vi "WPI_UtilitiesFRCAutomaticValuePublisher.vi"(11 "Enable":bool=TRUE) -> ()   [LabVIEW 2012]
uses:
  <vilib>/Rock Robotics/WPI/Utilities/Refnum Registry Operation.ctl
  <vilib>/Rock Robotics/WPI/Relay/WPI_RelayValue.ctl
  <vilib>/Rock Robotics/WPI/Solenoid/WPI_SolenoidValue.ctl
  <vilib>/Rock Robotics/WPI/Solenoid/WPI_SolenoidChannel.ctl
  <vilib>/Rock Robotics/WPI/Solenoid/WPI_SolenoidSetEnum.vi
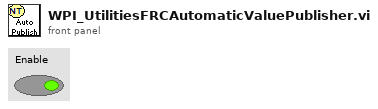
[diagram p1: front panel]
types:
  T1 = typedef "Refnum Registry Operation.ctl" = enum16{"set", "get", "delete", "get all names", "read name"}
  T2 = typedef "WPI_RelayValue.ctl" = enum16{"Off", "On", "Forward", "Reverse"}
  T3 = typedef "WPI_SolenoidChannel.ctl" = enum8{"Solenoid 1", "Solenoid 2", "Solenoid 3", "Solenoid 4", "Solenoid 5", "Solenoid 6", "Solenoid 7", "Solenoid 8", "Invalid"}
  T4 = typedef "WPI_SolenoidValue.ctl" = enum16{"Off", "On", "Forward", "Reverse"}
  T5 = typedef "WPI_JoystickDevRef.ctl" = cluster{"Device":T6}
  T6 = typedef "WPI_JoystickDeviceEnum.ctl" = enum16{"USB 1", "USB 2", "USB 3", "USB 4", "Kinect 1", "Kinect 2"}
  T7 = typedef "WPI_JoystickButtonState.ctl" = cluster{"Button 1":bool, "Button 2":bool, "Button 3":bool, "Button 4":bool, "Button 5":bool, "Button 6":bool, "Button 7":bool, "Button 8":bool, "Button 9":bool, "Button 10":bool, "Button 11":bool, "Button 12":bool}
  T8 = cluster{"axis 1 (x)":dbl, "axis 2 (y)":dbl, "axis 3 (throttle)":dbl, "axis 4":dbl, "axis 5":dbl, "axis 6":dbl}
  T9 = typedef "WPI_MotorControlDeviceRef.ctl" = cluster{"DeviceStatus":errorcluster, "Type":enum16{"PWM", "CAN"}, "PWM":cluster{"Digital Module":T10, "PWM Channel":T11, "DeadBand":T12}, "CAN":cluster{"Device Number":u8, "Control Mode":T13, "Semaphore":T14, "Max Vout":dbl}, "Invert":bool, "TransformRef":T15, "InvTransformRef":T15}
  T10 = typedef "FPGA_TypedefDigitalModule.ctl" = enum16{"Digital Module 1", "Digital Module 2"}
  T11 = typedef "FPGA_DIOPWMChannel.ctl" = enum8{"PWM 1", "PWM 2", "PWM 3", "PWM 4", "PWM 5", "PWM 6", "PWM 7", "PWM 8", "PWM 9", "PWM 10", "Invalid"}
  T12 = typedef "WPI_PWMDeadband.ctl" = cluster{"Name":string, "maxPositivePwm":i32, "minPositivePwm":i32, "centerPwm":i32, "maxNegativePwm":i32, "minNegativePwm":i32, "angularRange":u16}
  T13 = typedef "WPI_CANJaguar_ControlMode.ctl" = enum8{"Percent VBus", "Current", "Speed", "Position", "Voltage"}
  T14 = typedef "Semaphore RefNum" = refnum<k1>
  T15 = typedef "WPI_PWMTransform_ConPane.ctl" = refnum<vi>
  T16 = typedef "WPI_ServoDeviceRef.ctl" = cluster{"DeviceStatus":errorcluster, "Digital Module":T10, "PWM Channel":T11, "DeadBand":T12}
  T17 = typedef "WPI_RelayDevRef.ctl" = cluster{"DevStatus":errorcluster, "Relay Channel":T18, "Digital Module":T10, "Relay Direction":T19}
  T18 = typedef "FPGA_DIORelayChannel.ctl" = enum8{"Relay 1", "Relay 2", "Relay 3", "Relay 4", "Relay 5", "Relay 6", "Relay 7", "Relay 8", "Invalid"}
  T19 = typedef "WPI_RelayDirection.ctl" = enum16{"Both directions", "Forward only", "Reverse only"}
  T20 = typedef "WPI_CompressorDevRef.ctl" = cluster{"DevStatus":errorcluster, "DigitalInputDevRef":T21, "RelayDevRef":T17}
  T21 = typedef "WPI_DigitalInputDevRef.ctl" = cluster{"DevStatus":errorcluster, "DIO Channel":T22, "Digital Module":T10}
  T22 = typedef "FPGA_DIOChannel.ctl" = enum8{"DIO 1", "DIO 2", "DIO 3", "DIO 4", "DIO 5", "DIO 6", "DIO 7", "DIO 8", "DIO 9", "DIO 10", "DIO 11", "DIO 12", "DIO 13", "DIO 14", "Invalid"}
  T23 = typedef "WPI_SolenoidDevRef.ctl" = cluster{"DevStatus":errorcluster, "Solenoid Module":T24, "Forward Solenoid Channel":T3, "Reverse Solenoid Channel":T3}
  T24 = typedef "FPGA_TypedefSolenoidModule.ctl" = enum16{"Solenoid Module 1", "Solenoid Module 2"}
  T25 = typedef "WPI_AccelerometerDevRef.ctl" = cluster{"DevStatus":errorcluster, "Analog Module":T26, "Analog Channel":T27, "Scaling":T28}
  T26 = typedef "FPGA_TypedefAnalogModule.ctl" = enum16{"Analog Module 1", "Analog Module 2"}
  T27 = typedef "FPGA_AIChannel.ctl" = enum8{"AI 1", "AI 2", "AI 3", "AI 4", "AI 5", "AI 6", "AI 7", "AI 8", "Invalid"}
  T28 = typedef "WPI_AccelerometerScaling.ctl" = cluster{"Gain (VoltsPerG)":dbl, "Center Voltage":dbl}
  T29 = typedef "WPI_CounterDevRef.ctl" = cluster{"DevStatus":errorcluster, "CntIndex":T30}
  T30 = typedef "FPGA_CounterCtrSystemIndex.ctl" = enum8{"Ctr 0", "Ctr 1", "Ctr 2", "Ctr 3", "Ctr 4", "Ctr 5", "Ctr 6", "Ctr 7", "Invalid"}
  T31 = typedef "WPI_GyroDevRef.ctl" = cluster{"DevStatus":errorcluster, "Analog Module":T26, "Analog Channel":T27, "Offset":dbl, "Gain (VoltsPerDegree/Second)":dbl}
  T32 = typedef "WPI_UltrasonicDeviceRef.ctl" = cluster{"DevStatus":errorcluster, "Ping Digital Module":T10, "Echo Digital Module":T10, "Ping Channel":T22, "Echo Channel":T22, "CntIndex":T30}
  T33 = typedef "WPI_EncoderDevRef.ctl" = cluster{"DevStatus":errorcluster, "EncoderIndex":T34, "CounterIndex":T30, "DistancePerCount":dbl, "Decoding Type":T35}
  T34 = typedef "FPGA_EncoderIdx.ctl" = enum8{"Enc 0", "Enc 1", "Enc 2", "Enc 3", "Invalid"}
  T35 = typedef "WPI_EncoderType.ctl" = enum16{"1x", "2x", "4x"}
  T36 = typedef "WPI_DigitalOutputDevRef.ctl" = cluster{"Digital Module":T10, "DIO Channel":T22, "DevStatus":errorcluster}
  T37 = typedef "WPI_PWMDeviceRef.ctl" = cluster{"DeviceStatus":errorcluster, "Digital Module":T10, "PWM Channel":T11}
  T38 = typedef "WPI_AnalogChannelDevRef.ctl" = cluster{"DevStatus":errorcluster, "Analog Module":T26, "Analog Channel":T27}
  T39 = typedef "WPI_CameraDevRef.ctl" = cluster{"Camera Address":string, "CameraStatus":errorcluster, "Acquire Image Notifier":refnum<notifier>}
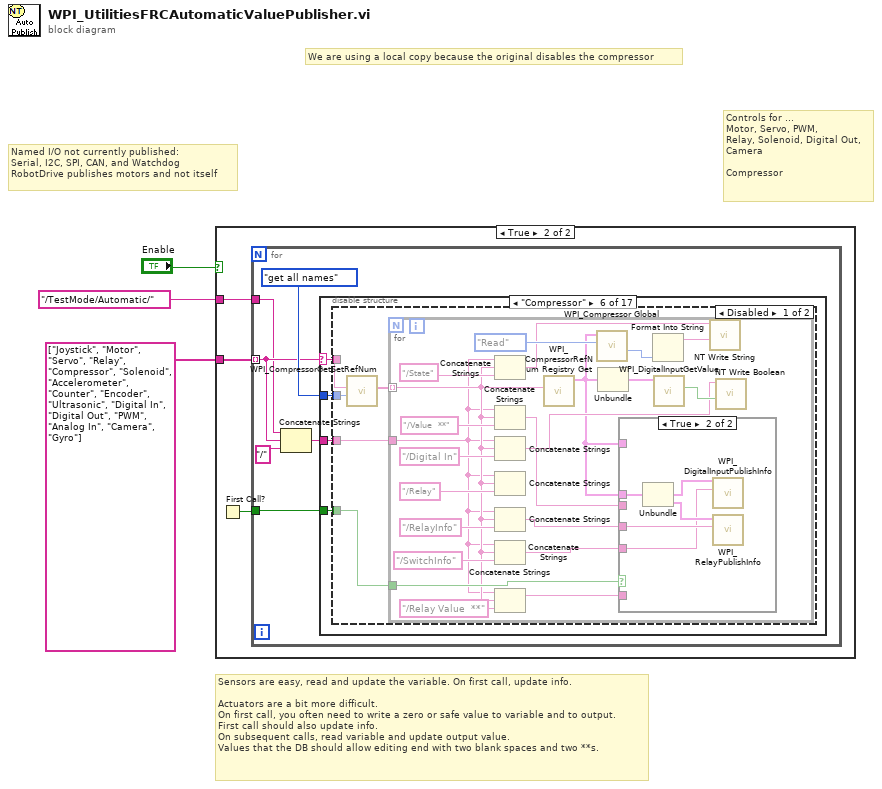
[diagram p0: block diagram]
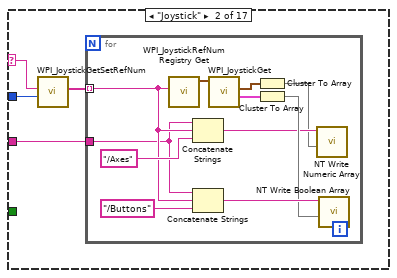
[diagram p4: hidden frame]
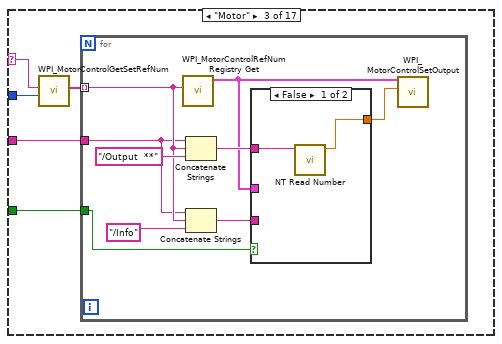
[diagram p5: hidden frame]
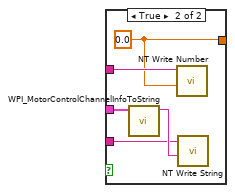
[diagram p6: hidden frame]
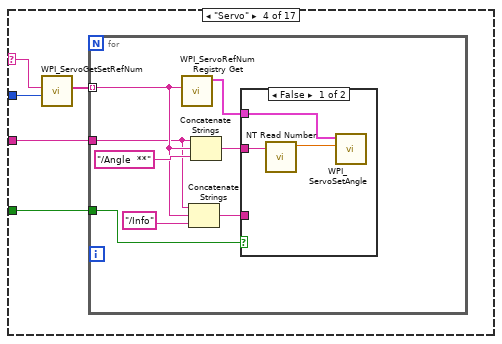
[diagram p7: hidden frame]
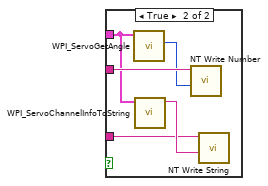
[diagram p8: hidden frame]
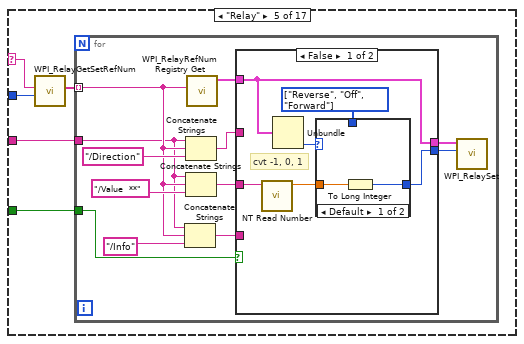
[diagram p9: hidden frame]
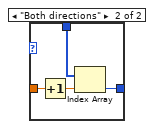
[diagram p10: hidden frame]
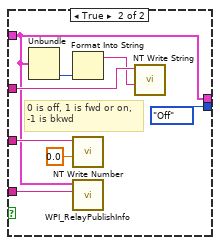
[diagram p11: hidden frame]
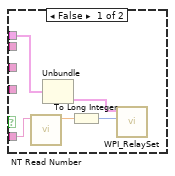
[diagram p12: hidden frame]
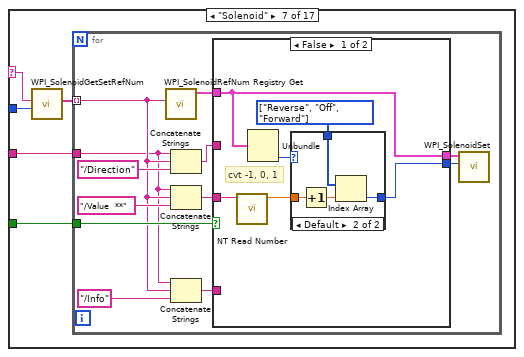
[diagram p14: hidden frame]
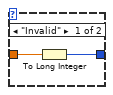
[diagram p15: hidden frame]
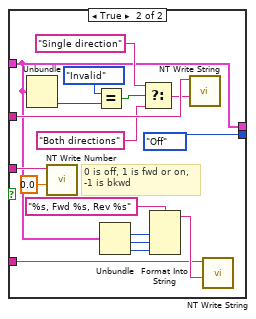
[diagram p16: hidden frame]
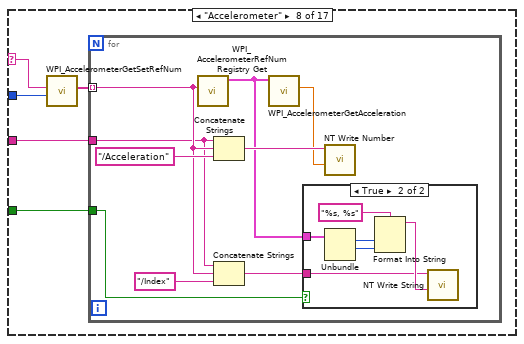
[diagram p17: hidden frame]
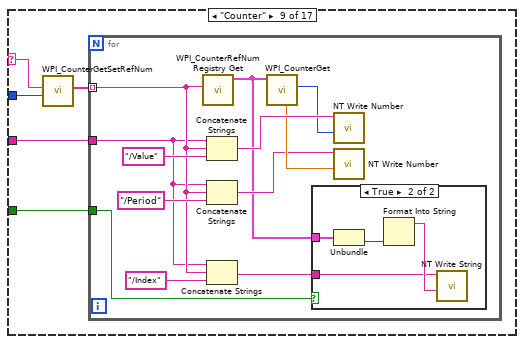
[diagram p19: hidden frame]
diagram:
  # "We are using a local copy because the original disables the compressor"
  # "Controls for ...\nMotor, Servo, PWM,\nRelay, Solenoid, Digital Out,\nCamera\n\nCompressor"
  # "Named I/O not currently published:\nSerial, I2C, SPI, CAN, and Watchdog\nRobotDrive publishes motors and not itself"
  # "Sensors are easy, read and update the variable. On first call, update info.\n\nActuators are a bit more difficult. \nOn first call, you often need to write a zero or safe value to variable and to output.\nFirst call should also update info.\nOn subsequent calls, read variable and update output value.\nValues that the DB should allow editing end with two blank spaces and two **s."
  n1 = case shown="True" "Enable" {
    tunnel: string[] ["Joystick", "Motor", "Servo", "Relay", "Compressor", "Solenoid", "Accelerometer", "Counter", "Encoder", "Ultrasonic", "Digital In", "Digital Out", "PWM", "Analog In", "Camera", "Gyro"] -> [_ w6]
    tunnel: "/TestMode/Automatic/" -> [_ w4]
    frame False {
    }
    frame True {
      n2 = First Call?() -> (First Call?: T/F=w5:bool)
      n3 = for {
        tunnel: w6 -> [w10] mode=indexing
        tunnel: w5 -> [w11]
        tunnel: w4 -> [w9]
        n4 = Concatenate Strings(w9, w10, "/") -> (w7:string)
        n5 = case shown="\"Compressor\"" w10 {
          selector: w10 -> [_ w14 w30 w50 w71 w108 w149 w196 w215 w236 w259 w282 w298 w322 w348 w373 w392]
          tunnel: Refnum_Registry_Operation."get all names" ("menu") -> [_ w15 w31 w51 w72 w109 w150 w195 w216 w237 w260 w283 w297 w323 w349 w372 w393]
          tunnel: w11 -> [_ _ w29 w53 w74 w110 w152 w198 w218 w239 w262 w285 w301 w325 w351 w375 w395]
          tunnel: w7 -> [_ w13 w28 w49 w70 w107 w148 w194 w214 w235 w258 w281 w300 w321 w347 w371 w391]
          frame Default {
            # "Unsupported I/O type"
          }
          frame "Joystick" {
            n6 = call <vilib>:"WPI_JoystickGetSetRefNum.vi"("menu"=w15, "refnum name"=w14) -> ("names"=w16:string[])  [unwired: 2 in, 7 out]
            n7 = for {
              tunnel: w16 -> [w18] mode=indexing
              tunnel: w13 -> [w17]
              n8 = call <vilib>:"WPI_JoystickRefNum Registry Get.vi"("refnum name"=w18) -> ("JoystickDevRef"=w27:T5)  [unwired: 9 in, 1 out]
              n9 = Concatenate Strings(w17, w18, "/Axes") -> (w21:string)
              n10 = Concatenate Strings(w17, w18, "/Buttons") -> (w25:string)
              n11 = call <vilib>:"WPI_JoystickGet.vi"("JoystickDevRef"=w27) -> ("Buttons"=w23:T7, "Axes"=w20:T8)  [unwired: 4 in, 1 out]
              n12 = Cluster To Array(cluster=w20) -> (array=w19:dbl[])
              n13 = Cluster To Array(cluster=w23) -> (array=w24:bool[])
              n14 = call <vilib>:"NT Write Numeric Array.vi"("Numeric Array"=w19, "Name"=w21) -> ()  [unwired: 9 in, 1 out]
              n15 = call <vilib>:"NT Write Boolean Array.vi"("Boolean Array"=w24, "Name"=w25) -> ()  [unwired: 9 in, 1 out]
            }
          }
          frame "Motor" {
            n16 = call <vilib>:"WPI_MotorControlGetSetRefNum.vi"("menu"=w31, "refnum name"=w30) -> ("refnum names"=w32:string[])  [unwired: 2 in, 7 out]
            n17 = for {
              tunnel: w32 -> [w36] mode=indexing
              tunnel: w29 -> [w38]
              tunnel: w28 -> [w35]
              n18 = call <vilib>:"WPI_MotorControlRefNum Registry Get.vi"("refnum name"=w36) -> ("MotorControlDevRef"=w34:T9)  [unwired: 9 in, 1 out]
              n19 = Concatenate Strings(w35, w36, "/Output  **") -> (w40:string)
              n20 = Concatenate Strings(w35, w36, "/Info") -> (w33:string)
              n21 = case shown="False" w38 {
                tunnel: w40 -> [w43 w48]
                tunnel: [w42 w47] -> w39
                tunnel: w34 -> [_ w45]
                tunnel: w33 -> [_ w44]
                frame False {
                  n22 = call <vilib>:"NT Read Number.vi"("Name"=w43) -> ("Numeric"=w42:dbl)  [unwired: 9 in, 1 out]
                }
                frame True {
                  w47 = 0.0
                  n23 = call <vilib>:"WPI_MotorControlChannelInfoToString.vi"("MotorControlDevRef"=w45) -> ("String"=w46:string)  [unwired: 10 in]
                  n24 = call <vilib>:"NT Write Number.vi"("Numeric"=w47, "Name"=w48) -> ()  [unwired: 9 in, 1 out]
                  n25 = call <vilib>:"NT Write String.vi"("String"=w46, "Name"=w44) -> ()  [unwired: 9 in, 1 out]
                }
              }
              n26 = call <vilib>:"WPI_MotorControlSetOutput.vi"("Output"=w39, "MotorControlDevRef"=w34) -> ()  [unwired: 7 in, 3 out]
            }
          }
          frame "Servo" {
            n27 = call <vilib>:"WPI_ServoGetSetRefNum.vi"("menu"=w51, "refnum name"=w50) -> ("names"=w52:string[])  [unwired: 7 in, 2 out]
            n28 = for {
              tunnel: w52 -> [w56] mode=indexing
              tunnel: w53 -> [w59]
              tunnel: w49 -> [w55]
              n29 = call <vilib>:"WPI_ServoRefNum Registry Get.vi"("refnum name"=w56) -> ("ServoDeviceRef"=w58:T16)  [unwired: 9 in, 1 out]
              n30 = Concatenate Strings(w55, w56, "/Info") -> (w54:string)
              n31 = Concatenate Strings(w55, w56, "/Angle  **") -> (w60:string)
              n32 = case shown="False" w59 {
                tunnel: w60 -> [w64 w69]
                tunnel: w58 -> [w62 w67]
                tunnel: w54 -> [_ w65]
                frame False {
                  n33 = call <vilib>:"NT Read Number.vi"("Name"=w64) -> ("Numeric"=w63:dbl)  [unwired: 9 in, 1 out]
                  n34 = call <vilib>:"WPI_ServoSetAngle.vi"("Angle"=w63, "ServoDeviceRef"=w62) -> ()  [unwired: 8 in, 2 out]
                }
                frame True {
                  n35 = call <vilib>:"WPI_ServoGetAngle.vi"("ServoDeviceRef"=w67) -> ("Angle"=w68:u16)  [unwired: 7 in, 2 out]
                  n36 = call <vilib>:"WPI_ServoChannelInfoToString.vi"("ServoDeviceRef"=w67) -> ("String"=w66:string)  [unwired: 10 in]
                  n37 = call <vilib>:"NT Write Number.vi"("Numeric"=w68, "Name"=w69) -> ()  [unwired: 9 in, 1 out]
                  n38 = call <vilib>:"NT Write String.vi"("String"=w66, "Name"=w65) -> ()  [unwired: 9 in, 1 out]
                }
              }
            }
          }
          frame "Relay" {
            n39 = call <vilib>:"WPI_RelayGetSetRefNum.vi"("menu"=w72, "refnum name"=w71) -> ("names"=w73:string[])  [unwired: 2 in, 7 out]
            n40 = for {
              tunnel: w73 -> [w77] mode=indexing
              tunnel: w74 -> [w84]
              tunnel: w70 -> [w76]
              n41 = Concatenate Strings(w76, w77, "/Info") -> (w75:string)
              n42 = Concatenate Strings(w76, w77, "/Direction") -> (w85:string)
              n43 = Concatenate Strings(w76, w77, "/Value  **") -> (w81:string)
              n44 = call <vilib>:"WPI_RelayRefNum Registry Get.vi"("refnum name"=w77) -> ("RelayDevRef"=w83:T17)  [unwired: 9 in, 1 out]
              n45 = case shown="False" w84 {
                tunnel: w85 -> [_ w106]
                tunnel: w83 -> [w88 w100]
                tunnel: w81 -> [w92 w102]
                tunnel: [w88 w100] -> w80
                tunnel: [w87 WPI_RelayValue."Off" ("RelayValue")] -> w79
                tunnel: w75 -> [_ w99]
                frame False {
                  w89 = T2[] [enum."Reverse", enum."Off", enum."Forward"] items=["Off", "On", "Forward", "Reverse"]
                  # "cvt -1, 0, 1"
                  n46 = call <vilib>:"NT Read Number.vi"("Name"=w92) -> ("Numeric"=w91:dbl)  [unwired: 9 in, 1 out]
                  n47 = Unbundle(w88) -> ("Relay Direction"=w90:T19)  [unwired: 3 out]
                  n48 = case shown="Default" w90 {
                    tunnel: w91 -> [w94 w98]
                    tunnel: w89 -> [_ w96]
                    tunnel: [w93 w95] -> w87
                    frame Default {
                      n49 = To Long Integer(number=w94) -> (32bit integer=w93:i32)
                    }
                    frame "Both directions" {
                      n50 = Increment(x=w98) -> (x+1=w97:dbl)
                      n51 = Index Array(array=w96, index=w97) -> (element=w95:T2)
                    }
                  }
                }
                frame True {
                  # "0 is off, 1 is fwd or on,\n-1 is bkwd"
                  n52 = Unbundle(w100) -> ("Relay Direction"=w104:T19)  [unwired: 3 out]
                  n53 = Format Into String(w104) -> (resulting string=w105:string)  [unwired: 3 in, 1 out]
                  n54 = call <vilib>:"NT Write Number.vi"("Numeric"=0.0, "Name"=w102) -> ()  [unwired: 9 in, 1 out]
                  n55 = call <vilib>:"WPI_RelayPublishInfo.vi"("Name"=w99, "RelayDevRef"=w100) -> ()  [unwired: 10 in]
                  n56 = call <vilib>:"NT Write String.vi"("String"=w105, "Name"=w106) -> ()  [unwired: 9 in, 1 out]
                }
              }
              n57 = call <vilib>:"WPI_RelaySet.vi"("RelayValue"=w79, "RelayDevRef"=w80) -> ()  [unwired: 8 in, 2 out]
            }
          }
          frame "Compressor" {
            n58 = disable-structure shown="Disabled" {
              disable-tunnel: w110 -> [w115 _]
              disable-tunnel: w109 -> [w113 _]
              disable-tunnel: w108 -> [w112 _]
              disable-tunnel: w107 -> [w111 _]
              frame Disabled {
                n59 = call <vilib>:"WPI_CompressorGetSetRefNum.vi"("menu"=w113, "refnum name"=w112) -> ("names"=w114:string[])  [unwired: 7 in, 2 out]
                n60 = for {
                  tunnel: w114 -> [w118] mode=indexing
                  tunnel: w115 -> [w129]
                  tunnel: w111 -> [w117]
                  n61 = Concatenate Strings(w117, w118, "/State") -> (w122:string)
                  n62 = Concatenate Strings(w117, w118, "/Value  **") -> (w120:string)
                  n63 = Concatenate Strings(w117, w118, "/Digital In") -> (w124:string)
                  n64 = Concatenate Strings(w117, w118, "/Relay") -> ()  [unwired: 1 out]
                  n65 = Concatenate Strings(w117, w118, "/RelayInfo") -> (w126:string)
                  n66 = Concatenate Strings(w117, w118, "/SwitchInfo") -> (w125:string)
                  n67 = Concatenate Strings(w117, w118, "/Relay Value  **") -> (w116:string)
                  n68 = call <vilib>:"WPI_CompressorRefNum Registry Get.vi"("refnum name"=w118) -> ("CompressorDevRef"=w123:T20)  [unwired: 9 in, 1 out]
                  n69 = call <vilib>:"WPI_Compressor Global.vi"("Operation"=enum16{"Read", "Write", "Add", "Remove"}."Read", "CompressorDevRef"=w123) -> ("Compressor State Out"=w132:enum16{"Disabled", "Running", "At Pressure"})  [unwired: 8 in, 1 out]
                  n70 = Unbundle(w123) -> ("DigitalInputDevRef"=w136:T21)  [unwired: 2 out]
                  n71 = case shown="True" w129 {
                    tunnel: w123 -> [w139 w147]
                    tunnel: w126 -> [_ w145]
                    tunnel: w125 -> [_ w143]
                    tunnel: w123 -> [_ _]
                    tunnel: w120 -> [_ _]
                    tunnel: w116 -> [w142 _]
                    frame False {
                      n72 = call <vilib>:"NT Read Number.vi"("Name"=w142) -> ("Numeric"=w140:dbl)  [unwired: 9 in, 1 out]
                      n73 = Unbundle(w139) -> ("RelayDevRef"=w138:T17)  [unwired: 2 out]
                      n74 = To Long Integer(number=w140) -> (32bit integer=w141:i32)
                      n75 = call <vilib>:"WPI_RelaySet.vi"("RelayValue"=w141, "RelayDevRef"=w138) -> ()  [unwired: 8 in, 2 out]
                    }
                    frame True {
                      n76 = Unbundle(w147) -> ("DigitalInputDevRef"=w144:T21, "RelayDevRef"=w146:T17)  [unwired: 1 out]
                      n77 = call <vilib>:"WPI_DigitalInputPublishInfo.vi"("Name"=w143, "DigitalInputDevRef"=w144) -> ()  [unwired: 10 in]
                      n78 = call <vilib>:"WPI_RelayPublishInfo.vi"("Name"=w145, "RelayDevRef"=w146) -> ()  [unwired: 10 in]
                    }
                  }
                  n79 = Format Into String(w132) -> (resulting string=w131:string)  [unwired: 3 in, 1 out]
                  n80 = call <vilib>:"WPI_DigitalInputGetValue.vi"("DigitalInputDevRef"=w136) -> ("Value"=w135:bool)  [unwired: 8 in, 2 out]
                  n81 = call <vilib>:"NT Write String.vi"("String"=w131, "Name"=w122) -> ()  [unwired: 9 in, 1 out]
                  n82 = call <vilib>:"NT Write Boolean.vi"("Boolean"=w135, "Name"=w124) -> ()  [unwired: 9 in, 1 out]
                }
              }
              frame Enabled {
              }
            }
          }
          frame "Solenoid" {
            n83 = call <vilib>:"WPI_SolenoidGetSetRefNum.vi"("menu"=w150, "refnum name"=w149) -> ("names"=w151:string[])  [unwired: 7 in, 2 out]
            n84 = for {
              tunnel: w151 -> [w155] mode=indexing
              tunnel: w152 -> [w160]
              tunnel: w148 -> [w154]
              n85 = call <vilib>:"WPI_SolenoidRefNum Registry Get.vi"("refnum name"=w155) -> ("SolenoidDevRef"=w157:T23)  [unwired: 9 in, 1 out]
              n86 = Concatenate Strings(w154, w155, "/Direction") -> (w163:string)
              n87 = Concatenate Strings(w154, w155, "/Value  **") -> (w158:string)
              n88 = Concatenate Strings(w154, w155, "/Info") -> (w153:string)
              n89 = case shown="False" w160 {
                tunnel: w163 -> [_ w193]
                tunnel: w157 -> [w167 w178]
                tunnel: w158 -> [w170 w191]
                tunnel: [w167 w178] -> w162
                tunnel: [w166 WPI_SolenoidValue."Off" ("Relay Value")] -> w161
                tunnel: w153 -> [_ w180]
                frame False {
                  w168 = T4[] [enum."Reverse", enum."Off", enum."Forward"] items=["Off", "On", "Forward", "Reverse"]
                  # "cvt -1, 0, 1"
                  n90 = call <vilib>:"NT Read Number.vi"("Name"=w170) -> ("Numeric"=w169:dbl)  [unwired: 9 in, 1 out]
                  n91 = Unbundle(w167) -> ("Reverse Solenoid Channel"=w165:T3)  [unwired: 3 out]
                  n92 = case shown="Default" w165 {
                    tunnel: w169 -> [w172 w176]
                    tunnel: w168 -> [_ w174]
                    tunnel: [w171 w173] -> w166
                    frame "Invalid" {
                      n93 = To Long Integer(number=w172) -> (32bit integer=w171:i32)
                    }
                    frame Default {
                      n94 = Increment(x=w176) -> (x+1=w175:dbl)
                      n95 = Index Array(array=w174, index=w175) -> (element=w173:T4)
                    }
                  }
                }
                frame True {
                  # "0 is off, 1 is fwd or on,\n-1 is bkwd"
                  n96 = Unbundle(w178) -> ("Reverse Solenoid Channel"=w189:T3)  [unwired: 3 out]
                  n97 = call <vilib>:"NT Write Number.vi"("Numeric"=0.0, "Name"=w191) -> ()  [unwired: 9 in, 1 out]
                  n98 = Equal?(x=WPI_SolenoidChannel."Invalid" ("Reverse Solenoid Channel"), y=w189) -> (x = y?=w188:bool)
                  n99 = Unbundle(w178) -> ("Solenoid Module"=w181:T24, "Forward Solenoid Channel"=w182:T3, "Reverse Solenoid Channel"=w177:T3)  [unwired: 1 out]
                  n100 = Select(t="Single direction", s=w188, f="Both directions") -> (s? t:f=w184:string)
                  n101 = Format Into String(format string="%s, Fwd %s, Rev %s", w181, w182, w177) -> (resulting string=w183:string)  [unwired: 2 in, 1 out]
                  n102 = call <vilib>:"NT Write String.vi"("String"=w184, "Name"=w193) -> ()  [unwired: 9 in, 1 out]
                  n103 = call <vilib>:"NT Write String.vi"("String"=w183, "Name"=w180) -> ()  [unwired: 9 in, 1 out]
                }
              }
              n104 = call-poly <vilib>:"WPI_SolenoidSet.vi"("Value"=w161, "SolenoidDevRef"=w162) -> ()  [unwired: 8 in, 2 out]
            }
          }
          frame "Accelerometer" {
            n105 = call <vilib>:"WPI_AccelerometerGetSetRefNum.vi"("menu"=w195, "refnum name"=w196) -> ("refnum names"=w197:string[])  [unwired: 7 in, 2 out]
            n106 = for {
              tunnel: w197 -> [w203] mode=indexing
              tunnel: w198 -> [w201]
              tunnel: w194 -> [w202]
              n107 = call <vilib>:"WPI_AccelerometerRefNum Registry Get.vi"("refnum name"=w203) -> ("AccelerometerDevRef"=w200:T25)  [unwired: 9 in, 1 out]
              n108 = Concatenate Strings(w202, w203, "/Acceleration") -> (w206:string)
              n109 = Concatenate Strings(w202, w203, "/Index") -> (w199:string)
              n110 = call <vilib>:"WPI_AccelerometerGetAcceleration.vi"("AccelerometerDevRef"=w200) -> ("Acceleration"=w205:dbl)  [unwired: 8 in, 2 out]
              n111 = case shown="True" w201 {
                tunnel: w199 -> [_ w208]
                tunnel: w200 -> [_ w213]
                frame False {
                }
                frame True {
                  n112 = Unbundle(w213) -> ("Analog Module"=w212:T26, "Analog Channel"=w211:T27)  [unwired: 2 out]
                  n113 = Format Into String(format string="%s, %s", w212, w211) -> (resulting string=w209:string)  [unwired: 2 in, 1 out]
                  n114 = call <vilib>:"NT Write String.vi"("String"=w209, "Name"=w208) -> ()  [unwired: 9 in, 1 out]
                }
              }
              n115 = call <vilib>:"NT Write Number.vi"("Numeric"=w205, "Name"=w206) -> ()  [unwired: 9 in, 1 out]
            }
          }
          frame "Counter" {
            n116 = call <vilib>:"WPI_CounterGetSetRefNum.vi"("menu"=w216, "refnum name"=w215) -> ("refnum names"=w217:string[])  [unwired: 2 in, 7 out]
            n117 = for {
              tunnel: w217 -> [w221] mode=indexing
              tunnel: w218 -> [w219]
              tunnel: w214 -> [w220]
              n118 = call <vilib>:"WPI_CounterRefNum Registry Get.vi"("refnum name"=w221) -> ("CounterDevRef"=w224:T29)  [unwired: 9 in, 1 out]
              n119 = Concatenate Strings(w220, w221, "/Value") -> (w229:string)
              n120 = Concatenate Strings(w220, w221, "/Period") -> (w225:string)
              n121 = Concatenate Strings(w220, w221, "/Index") -> (w222:string)
              n122 = call <vilib>:"WPI_CounterGet.vi"("CounterDevRef in"=w224) -> ("Value"=w228:i32, "Period (sec)"=w227:dbl)  [unwired: 5 in, 4 out]
              n123 = case shown="True" w219 {
                tunnel: w222 -> [_ w231]
                tunnel: w224 -> [_ w234]
                frame False {
                }
                frame True {
                  n124 = Unbundle(w234) -> ("CntIndex"=w233:T30)  [unwired: 1 out]
                  n125 = Format Into String(w233) -> (resulting string=w232:string)  [unwired: 3 in, 1 out]
                  n126 = call <vilib>:"NT Write String.vi"("String"=w232, "Name"=w231) -> ()  [unwired: 9 in, 1 out]
                }
              }
              n127 = call <vilib>:"NT Write Number.vi"("Numeric"=w228, "Name"=w229) -> ()  [unwired: 9 in, 1 out]
              n128 = call <vilib>:"NT Write Number.vi"("Numeric"=w227, "Name"=w225) -> ()  [unwired: 9 in, 1 out]
            }
          }
          frame "Gyro" {
            n129 = call <vilib>:"WPI_GyroGetSetRefNum.vi"("menu"=w237, "refnum name"=w236) -> ("refnum names"=w238:string[])  [unwired: 2 in, 7 out]
            n130 = for {
              tunnel: w238 -> [w243] mode=indexing
              tunnel: w239 -> [w240]
              tunnel: w235 -> [w242]
              n131 = call <vilib>:"WPI_GyroRefNum Registry Get.vi"("refnum name"=w243) -> ("GyroDevRef"=w245:T31)  [unwired: 9 in, 1 out]
              n132 = Concatenate Strings(w242, w243, "/Angle") -> (w250:string)
              n133 = Concatenate Strings(w242, w243, "/Rate") -> (w248:string)
              n134 = Concatenate Strings(w242, w243, "/Info") -> (w241:string)
              n135 = call <vilib>:"WPI_GyroGetAngle.vi"("GyroDevRef"=w245) -> ("Angular Rate"=w246:dbl, "Angle"=w247:dbl)  [unwired: 7 in, 2 out]
              n136 = case shown="True" w240 {
                tunnel: w241 -> [_ w252]
                tunnel: w245 -> [_ w257]
                frame False {
                }
                frame True {
                  n137 = Unbundle(w257) -> ("Analog Module"=w256:T26, "Analog Channel"=w255:T27)  [unwired: 3 out]
                  n138 = Format Into String(format string="%s, %s", w256, w255) -> (resulting string=w253:string)  [unwired: 2 in, 1 out]
                  n139 = call <vilib>:"NT Write String.vi"("String"=w253, "Name"=w252) -> ()  [unwired: 9 in, 1 out]
                }
              }
              n140 = call <vilib>:"NT Write Number.vi"("Numeric"=w247, "Name"=w250) -> ()  [unwired: 9 in, 1 out]
              n141 = call <vilib>:"NT Write Number.vi"("Numeric"=w246, "Name"=w248) -> ()  [unwired: 9 in, 1 out]
            }
          }
          frame "Ultrasonic" {
            n142 = call <vilib>:"WPI_UltrasonicGetSetRefNum.vi"("menu"=w260, "refnum name"=w259) -> ("names"=w261:string[])  [unwired: 7 in, 2 out]
            n143 = for {
              tunnel: w261 -> [w268] mode=indexing
              tunnel: w262 -> [w263]
              tunnel: w258 -> [w267]
              n144 = call <vilib>:"WPI_UltrasonicRefNum Registry Get.vi"("refnum name"=w268) -> ("UltrasonicDevRef"=w265:T32)  [unwired: 9 in, 1 out]
              n145 = Concatenate Strings(w267, w268, "/Distance") -> (w271:string)
              n146 = Concatenate Strings(w267, w268, "/Info") -> (w266:string)
              n147 = call <vilib>:"WPI_UltrasonicGetRange.vi"("UltrasonicDevRef"=w265) -> ("Distance"=w270:dbl)  [unwired: 8 in, 2 out]
              n148 = case shown="True" w263 {
                tunnel: w266 -> [_ w277]
                tunnel: w265 -> [_ w280]
                tunnel: "Ping %s, %s; Echo %s, %s" ("format string") -> [_ w273]
                frame False {
                }
                frame True {
                  n149 = Unbundle(w280) -> ("Ping Digital Module"=w279:T10, "Echo Digital Module"=w274:T10, "Ping Channel"=w276:T22, "Echo Channel"=w275:T22)  [unwired: 2 out]
                  n150 = Format Into String(format string=w273, w279, w276, w274, w275) -> (resulting string=w278:string)  [unwired: 2 in, 1 out]
                  n151 = call <vilib>:"NT Write String.vi"("String"=w278, "Name"=w277) -> ()  [unwired: 9 in, 1 out]
                }
              }
              n152 = call <vilib>:"NT Write Number.vi"("Numeric"=w270, "Name"=w271) -> ()  [unwired: 9 in, 1 out]
            }
          }
          frame "Digital In" {
            n153 = call <vilib>:"WPI_DigitalInputGetSetRefNum.vi"("menu"=w283, "refnum name"=w282) -> ("names"=w284:string[])  [unwired: 2 in, 7 out]
            n154 = for {
              tunnel: w284 -> [w289] mode=indexing
              tunnel: w285 -> [w290]
              tunnel: w281 -> [w288]
              n155 = Concatenate Strings(w288, w289, "/Value") -> (w293:string)
              n156 = Concatenate Strings(w288, w289, "/Info") -> (w287:string)
              n157 = call <vilib>:"WPI_DigitalInputRefNum Registry Get.vi"("refnum name"=w289) -> ("DigitalInputDevRef"=w286:T21)  [unwired: 9 in, 1 out]
              n158 = case shown="True" w290 {
                tunnel: w287 -> [_ w295]
                tunnel: w286 -> [_ w296]
                frame False {
                }
                frame True {
                  n159 = call <vilib>:"WPI_DigitalInputPublishInfo.vi"("Name"=w295, "DigitalInputDevRef"=w296) -> ()  [unwired: 10 in]
                }
              }
              n160 = call <vilib>:"WPI_DigitalInputGetValue.vi"("DigitalInputDevRef"=w286) -> ("Value"=w292:bool)  [unwired: 8 in, 2 out]
              n161 = call <vilib>:"NT Write Boolean.vi"("Boolean"=w292, "Name"=w293) -> ()  [unwired: 9 in, 1 out]
            }
          }
          frame "Encoder" {
            n162 = call <vilib>:"WPI_EncoderGetSetRefNum.vi"("menu"=w297, "refnum name"=w298) -> ("refnum names"=w299:string[])  [unwired: 2 in, 7 out]
            n163 = for {
              tunnel: w299 -> [w302] mode=indexing
              tunnel: w301 -> [w311]
              tunnel: w300 -> [w303]
              n164 = Concatenate Strings(w303, w302, "/Distance") -> (w308:string)
              n165 = Concatenate Strings(w303, w302, "/Rate") -> (w305:string)
              n166 = Concatenate Strings(w303, w302, "/Info") -> (w310:string)
              n167 = call <vilib>:"WPI_EncoderRefNum Registry Get.vi"("refnum name"=w302) -> ("EncoderDevRef"=w309:T33)  [unwired: 9 in, 1 out]
              n168 = case shown="True" w311 {
                tunnel: w310 -> [_ w317]
                tunnel: w309 -> [_ w314]
                frame False {
                }
                frame True {
                  n169 = Unbundle(w314) -> ("EncoderIndex"=w315:T34, "CounterIndex"=w320:T30, "Decoding Type"=w316:T35)  [unwired: 2 out]
                  n170 = call <vilib>:"WPI_EncoderStart.vi"("EncoderDevRef"=w314) -> ()  [unwired: 9 in, 2 out]
                  n171 = Format Into String(format string="%s, %s, %s", w316, w315, w320) -> (resulting string=w318:string)  [unwired: 2 in, 1 out]
                  n172 = call <vilib>:"NT Write String.vi"("String"=w318, "Name"=w317) -> ()  [unwired: 9 in, 1 out]
                }
              }
              n173 = call <vilib>:"WPI_EncoderGet.vi"("EncoderDevRef"=w309) -> ("Distance"=w307:dbl, "Rate"=w304:dbl)  [unwired: 5 in, 4 out]
              n174 = call <vilib>:"NT Write Number.vi"("Numeric"=w307, "Name"=w308) -> ()  [unwired: 9 in, 1 out]
              n175 = call <vilib>:"NT Write Number.vi"("Numeric"=w304, "Name"=w305) -> ()  [unwired: 9 in, 1 out]
            }
          }
          frame "Digital Out" {
            n176 = call <vilib>:"WPI_DigitalOutputGetSetRefNum.vi"("menu"=w323, "refnum name"=w322) -> ("names"=w324:string[])  [unwired: 2 in, 7 out]
            n177 = for {
              tunnel: w322 -> [_]
              tunnel: w324 -> [w328] mode=indexing
              tunnel: w325 -> [w331]
              tunnel: w321 -> [w327]
              n178 = call <vilib>:"WPI_DigitalOutputRefNum Registry Get.vi"("refnum name"=w328) -> ("DigitalOutputDevRef"=w330:T36)  [unwired: 9 in, 1 out]
              n179 = Concatenate Strings(w327, w328, "/Value  **") -> (w332:string)
              n180 = Concatenate Strings(w327, w328, "/Info") -> (w326:string)
              n181 = case shown="False" w331 {
                tunnel: w332 -> [w336 w339]
                tunnel: w330 -> [w337 w342]
                tunnel: w326 -> [_ w343]
                frame False {
                  n182 = call <vilib>:"NT Read Number.vi"("Name"=w336) -> ("Numeric"=w335:dbl)  [unwired: 9 in, 1 out]
                  n183 = Not Equal To 0?(x=w335) -> (x != 0?=w334:bool)
                  n184 = call <vilib>:"WPI_DigitalOutputSetValue.vi"("Value"=w334, "DigitalOutputDevRef"=w337) -> ()  [unwired: 8 in, 2 out]
                }
                frame True {
                  n185 = Unbundle(w342) -> ("Digital Module"=w341:T10, "DIO Channel"=w340:T22)  [unwired: 1 out]
                  n186 = Format Into String(format string="%s, %s", w341, w340) -> (resulting string=w345:string)  [unwired: 2 in, 1 out]
                  n187 = call <vilib>:"NT Write Number.vi"("Numeric"=0, "Name"=w339) -> ()  [unwired: 9 in, 1 out]
                  n188 = call <vilib>:"WPI_DigitalOutputSetValue.vi"("Value"=FALSE, "DigitalOutputDevRef"=w342) -> ()  [unwired: 8 in, 2 out]
                  n189 = call <vilib>:"NT Write String.vi"("String"=w345, "Name"=w343) -> ()  [unwired: 9 in, 1 out]
                }
              }
            }
          }
          frame "PWM" {
            n190 = call <vilib>:"WPI_PWMGetSetRefNum.vi"("menu"=w349, "refnum name"=w348) -> ("names"=w350:string[])  [unwired: 2 in, 7 out]
            n191 = for {
              tunnel: w350 -> [w355] mode=indexing
              tunnel: w351 -> [w358]
              tunnel: w347 -> [w354]
              n192 = call <vilib>:"WPI_PWMRefNum Registry Get.vi"("refnum name"=w355) -> ("PWMDeviceRef"=w353:T37)  [unwired: 9 in, 1 out]
              n193 = Concatenate Strings(w354, w355, "/Value  **") -> (w359:string)
              n194 = Concatenate Strings(w354, w355, "/Info") -> (w352:string)
              n195 = case shown="True" w358 {
                tunnel: w359 -> [w362 w370]
                tunnel: [w361 w369] -> w357
                tunnel: w353 -> [_ w364]
                tunnel: w352 -> [_ w363]
                frame False {
                  n196 = call <vilib>:"NT Read Number.vi"("Name"=w362) -> ("Numeric"=w361:dbl)  [unwired: 9 in, 1 out]
                }
                frame True {
                  w369 = u8 0 ("Value")
                  n197 = Unbundle(w364) -> ("Digital Module"=w365:T10, "PWM Channel"=w366:T11)  [unwired: 1 out]
                  n198 = call <vilib>:"NT Write Number.vi"("Numeric"=w369, "Name"=w370) -> ()  [unwired: 9 in, 1 out]
                  n199 = Format Into String(format string="%s, %s", w365, w366) -> (resulting string=w368:string)  [unwired: 2 in, 1 out]
                  n200 = call <vilib>:"NT Write String.vi"("String"=w368, "Name"=w363) -> ()  [unwired: 9 in, 1 out]
                }
              }
              n201 = call <vilib>:"WPI_PWMSetValue.vi"("Value"=w357, "PWMDeviceRef"=w353) -> ()  [unwired: 8 in, 2 out]
            }
          }
          frame "Analog In" {
            n202 = call <vilib>:"WPI_AnalogChannelGetSetRefNum.vi"("menu"=w372, "refnum name"=w373) -> ("names"=w374:string[])  [unwired: 2 in, 7 out]
            n203 = for {
              tunnel: w374 -> [w379] mode=indexing
              tunnel: w375 -> [w381]
              tunnel: w371 -> [w378]
              n204 = call <vilib>:"WPI_AnalogChannelRefNum Registry Get.vi"("refnum name"=w379) -> ("AIDeviceRef"=w376:T38)  [unwired: 9 in, 1 out]
              n205 = Concatenate Strings(w378, w379, "/Voltage") -> (w383:string)
              n206 = Concatenate Strings(w378, w379, "/Info") -> (w377:string)
              n207 = case shown="True" w381 {
                tunnel: w377 -> [_ w385]
                tunnel: w376 -> [_ w390]
                frame False {
                }
                frame True {
                  n208 = Unbundle(w390) -> ("Analog Module"=w389:T26, "Analog Channel"=w388:T27)  [unwired: 1 out]
                  n209 = Format Into String(format string="%s, %s", w389, w388) -> (resulting string=w386:string)  [unwired: 2 in, 1 out]
                  n210 = call <vilib>:"NT Write String.vi"("String"=w386, "Name"=w385) -> ()  [unwired: 9 in, 1 out]
                }
              }
              n211 = call <vilib>:"WPI_AnalogChannelGetVoltage.vi"("AIDeviceRef"=w376) -> ("Voltage"=w382:dbl)  [unwired: 8 in, 2 out]
              n212 = call <vilib>:"NT Write Number.vi"("Numeric"=w382, "Name"=w383) -> ()  [unwired: 9 in, 1 out]
            }
          }
          frame "Camera" {
            n213 = call <vilib>:"WPI_CameraGetSetRefNum.vi"("menu"=w393, "refnum name"=w392) -> ("names"=w394:string[])  [unwired: 2 in, 7 out]
            n214 = for {
              tunnel: w394 -> [w396] mode=indexing
              tunnel: w395 -> [w398]
              tunnel: w391 -> [w397]
              n215 = call <vilib>:"WPI_CameraRefNum Registry Get.vi"("refnum name"=w396) -> ("CameraDevRef"=w399:T39)  [unwired: 9 in, 1 out]
              n216 = case shown="False" w398 {
                tunnel: w399 -> [w402 w405]
                tunnel: w397 -> [w401 w404]
                tunnel: w396 -> [w400 w403]
                frame False {
                  n217 = call <vilib>:"WPI_CameraUpdate Settings.vi"("Name"=w400, "Table"=w401, "CameraDevRef"=w402) -> ()  [unwired: 9 in]
                }
                frame True {
                  n218 = call <vilib>:"WPI_CameraPublish Settings.vi"("Name"=w403, "Table"=w404, "CameraDevRef"=w405) -> ()  [unwired: 9 in]
                }
              }
            }
          }
        }
      }
    }
  }
